vi "LJUD_ResetLabJack.vi"(8 "error in":errorcluster, 10 "Soft Reset Only":bool, 11 "Handle In":i32) -> (0 "error out":errorcluster, 3 "Handle Out":i32)   [LabVIEW 2021]
doc: "Sends a reset command to the LabJack hardware. Reset causes\nthe device to go to the reset/power-up configuration.\n\nDocumented in Section 4.2 of the device's datasheet."
uses:
  labjackud.dll
panel:
  # "Sends a reset command to the LabJack hardware. Reset causes\nthe device to go to the reset/power-up configuration.\n\nDocumented in Section 4.2 of the device's datasheet."
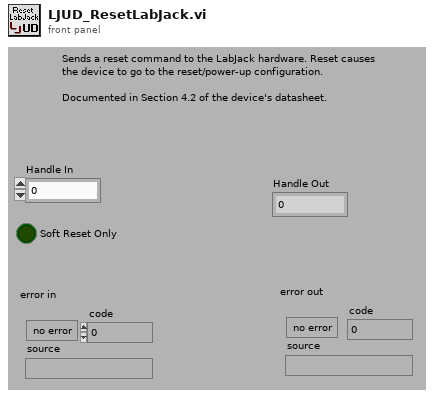
[diagram p1: front panel]
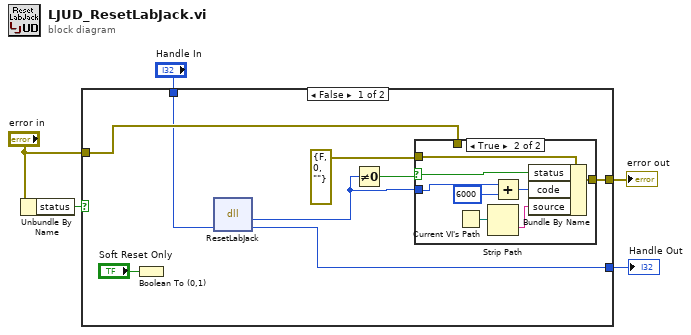
[diagram p0: block diagram]
diagram:
  n1 = Unbundle By Name("error in") -> ("status"=w3:bool)
  n2 = case shown="False" w3 {
    tunnel: [w11 w24] -> w5
    tunnel: "error in" -> [w8 w24]
    tunnel: "Handle In" -> [w7 w23]
    tunnel: [w6 w23] -> w1
    frame False {
      n3 = Boolean To (0,1)(Boolean="Soft Reset Only") -> ()  [unwired: 1 out]
      n4 = dll-call lib="labjackud.dll" fn="ResetLabJack"("Handle"=w7) -> (w12:i32, "Handle"=w6:i32)  [unwired: 3 in, 2 out]
      n5 = Not Equal To 0?(x=w12) -> (x != 0?=w10:bool)
      n6 = case shown="True" w10 {
        selector: w10 -> [_ w21]
        tunnel: [w14 w22] -> w11
        tunnel: errorcluster {"status"=FALSE, "code"=0, "source"=""} ("error IO") -> [_ w20]
        tunnel: w12 -> [_ w16]
        tunnel: w8 -> [w14 _]
        frame False {
        }
        frame True {
          n7 = Current VI's Path() -> (path=w18:path)
          n8 = Strip Path(path=w18) -> (name=w19:string)  [unwired: 1 out]
          n9 = Add(x=w16, y=6000) -> (x+y=w17:i32)
          n10 = Bundle By Name(cluster=w20, "status"=w21, "code"=w17, "source"=w19) -> (w22:errorcluster)
        }
      }
    }
    frame True {
    }
  }
  "error out" <- w5
  "Handle Out" <- w1
